vi "Tote Motor Update.vi"(10 "RelayDevRef 2":T1={"DevStatus"={"status"=FALSE, "code"=0, "source"=""}, "Relay Channel"=enum."Relay 1", "Relay Direction"=enum."Both directions"}, 11 "RelayDevRef":T1={"DevStatus"={"status"=FALSE, "code"=0, "source"=""}, "Relay Channel"=enum."Relay 1", "Relay Direction"=enum."Both directions"}) -> ()   [LabVIEW 2015]
uses:
  <vilib>/Rock Robotics/WPI/Relay/WPI_RelayDevRef.ctl
  <vilib>/Rock Robotics/SystemInterfaces/DIO/FPGA_DIORelayChannel.ctl
  <vilib>/Rock Robotics/WPI/Relay/WPI_RelayDirection.ctl
  Robot Values.vi
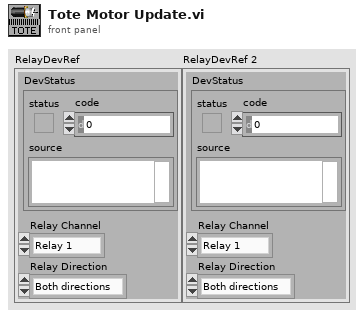
[diagram p1: front panel]
types:
  T1 = typedef "WPI_RelayDevRef.ctl" = cluster{"DevStatus":errorcluster, "Relay Channel":T2, "Relay Direction":T3}
  T2 = typedef "FPGA_DIORelayChannel.ctl" = enum8{"Relay 0", "Relay 1", "Relay 2", "Relay 3", "Invalid"}
  T3 = typedef "WPI_RelayDirection.ctl" = enum16{"Both directions", "Forward only", "Reverse only"}
  T4 = typedef "WPI_RelayValue.ctl" = enum16{"Off", "On", "Forward", "Reverse"}
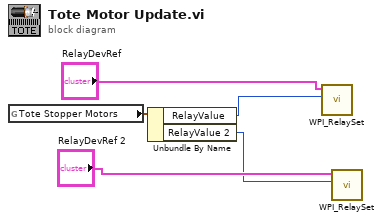
[diagram p0: block diagram]
diagram:
  n1 = global read "Robot Values.vi" "Tote Stopper Motors"() -> (w3:cluster{"RelayValue":T4, "RelayValue 2":T4})
  n2 = Unbundle By Name(w3) -> ("RelayValue"=w2:T4, "RelayValue 2"=w1:T4)
  n3 = call <vilib>:"WPI_RelaySet.vi"("RelayValue"=w2, "RelayDevRef"="RelayDevRef") -> ()  [unwired: 8 in, 2 out]
  n4 = call <vilib>:"WPI_RelaySet.vi"("RelayValue"=w1, "RelayDevRef"="RelayDevRef 2") -> ()  [unwired: 8 in, 2 out]
